vi "Write Default Rectangle Cluster.vi"(8 "error in (no error)":errorcluster, 10 "Default Rectangle":T1, 11 "Rectangle Settings in":refnum<class "Rectangle Settings.lvclass">) -> (0 "error out":errorcluster, 3 "Rectangle Settings out":refnum<class "Rectangle Settings.lvclass">)   [LabVIEW 2019, in "Rectangle Settings.lvclass"]
uses:
  Rectangle Settings.lvclass
  Typedefs/Default Rectangle Cluster.ctl
  Rectangle Settings.lvclass/Rectangle Settings.ctl
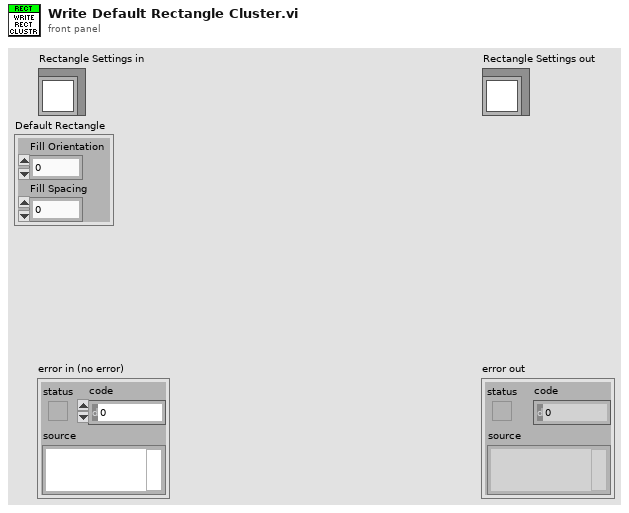
[diagram p1: front panel]
types:
  T1 = typedef "Rectangle Settings.lvclass/Default Rectangle Cluster.ctl" = cluster{"Fill Orientation":u16, "Fill Spacing":dbl}
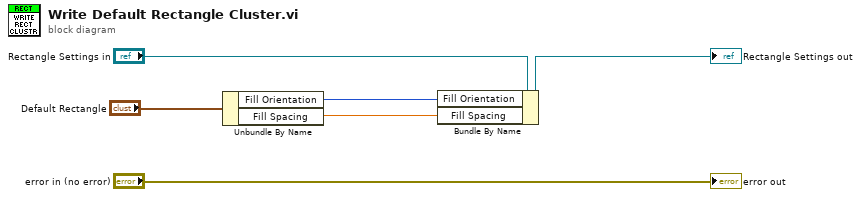
[diagram p0: block diagram]
diagram:
  n1 = Unbundle By Name("Default Rectangle") -> ("Fill Orientation"=w2:u16, "Fill Spacing"=w1:dbl)
  n2 = Bundle By Name(cluster="Rectangle Settings in", "Fill Orientation"=w2, "Fill Spacing"=w1) -> (→"Rectangle Settings out":refnum<class "Rectangle Settings.lvclass">)
  "error out" <- "error in (no error)"
